vi "generate_chirp_3326A.vi"() -> ()   [LabVIEW 2014]
panel:
  in  "Zero Offsets?":bool=TRUE
  in  "B: Phase (deg)":dbl format="%#_13g"
  in  "A: Phase (deg)":dbl format="%#_13g"
  in  "B: Offset Trim (part per thousand)":i32
  in  "B: Auto Offset":bool=TRUE
  in  "B: Manual Offset (V)":dbl=175.0
  in  "Desired Final Amplitude (V)":dbl format="%#_13g"
  in  "CH B Gain":dbl format="%#_13g"
  in  "CH A Gain":dbl format="%#_13g"
  in  "Step Length (s)":i32=10000
  in  "A: Offset Trim (part per thousand)":i32
  in  "A: Auto Offset":bool=TRUE
  in  "A: Manual Offset (V)":dbl=175.0
  in  "Hz/step":dbl=300.0
  out "Current Freq":dbl format="%#_13g"
  in  "Stop Freq (Hz)":dbl=300.0
  in  "Start Freq (Hz)":dbl=175.0
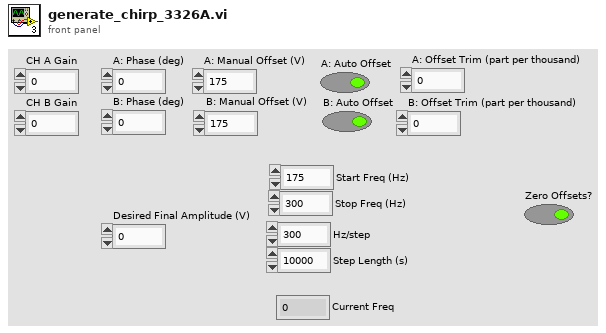
[diagram p1: front panel]
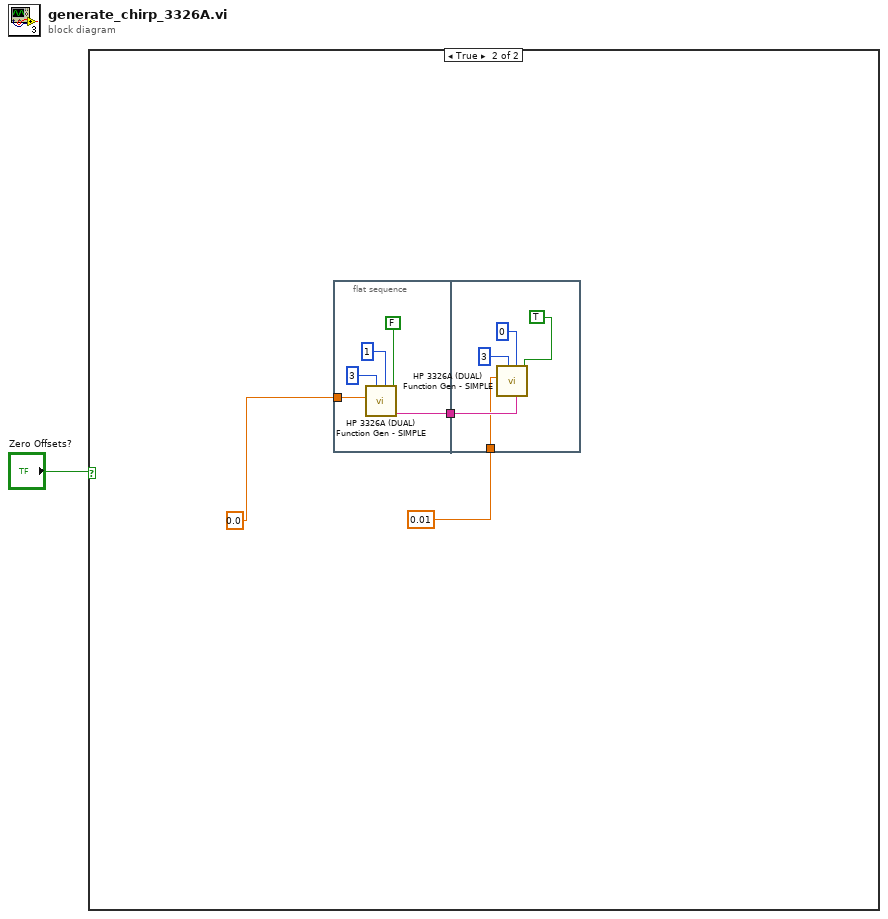
[diagram p0: block diagram]
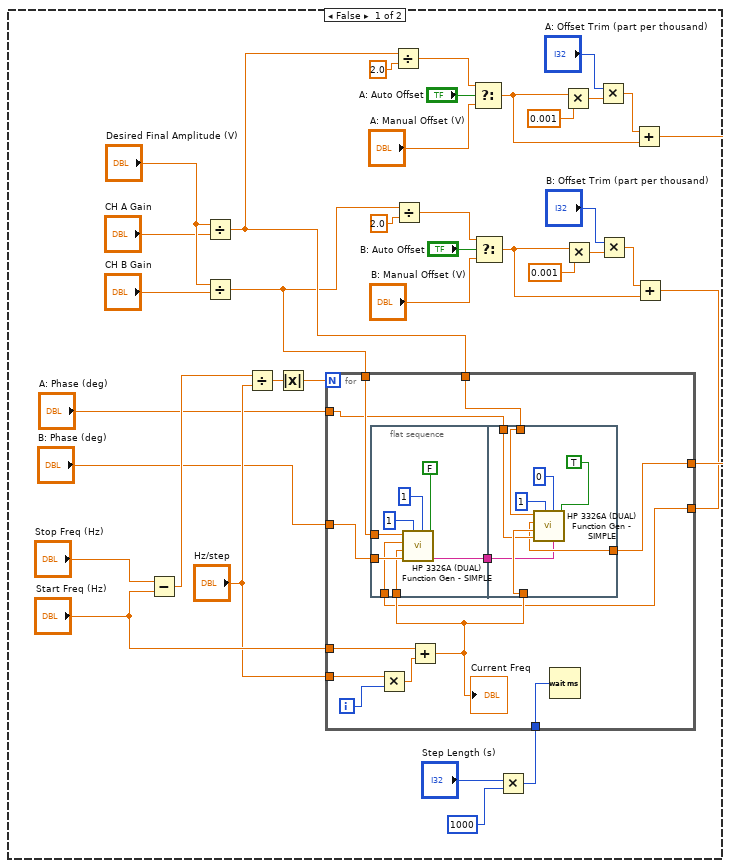
[diagram p2: hidden frame]
diagram:
  n1 = case shown="True" "Zero Offsets?" {
    frame False {
      n2 = Subtract(x="Stop Freq (Hz)", y="Start Freq (Hz)") -> (x-y=w36:dbl)
      n3 = Divide(x="Desired Final Amplitude (V)", y="CH A Gain") -> (x/y=w7:dbl)
      n4 = Divide(x="Desired Final Amplitude (V)", y="CH B Gain") -> (x/y=w6:dbl)
      n5 = Divide(x=w36, y="Hz/step") -> (x/y=w21:dbl)
      n6 = Absolute Value(x=w21) -> (abs(x)=w20:dbl)
      n7 = Divide(x=w7, y=2.0) -> (x/y=w32:dbl)
      n8 = Divide(x=w6, y=2.0) -> (x/y=w14:dbl)
      n9 = Select(t=w32, s="A: Auto Offset", f="A: Manual Offset (V)") -> (s? t:f=w30:dbl)
      n10 = Select(t=w14, s="B: Auto Offset", f="B: Manual Offset (V)") -> (s? t:f=w12:dbl)
      n11 = Multiply(x="Step Length (s)", y=1000) -> (x*y=w22:i32)
      n12 = Multiply(x=w30, y=0.001) -> (x*y=w27:dbl)
      n13 = Multiply(x=w12, y=0.001) -> (x*y=w9:dbl)
      n14 = Multiply(x="A: Offset Trim (part per thousand)", y=w27) -> (x*y=w26:dbl)
      n15 = Multiply(x="B: Offset Trim (part per thousand)", y=w9) -> (x*y=w8:dbl)
      n16 = Add(x=w26, y=w30) -> (x+y=w5:dbl)
      n17 = Add(x=w8, y=w12) -> (x+y=w4:dbl)
      n18 = for {
        N: w20 -> [_]
        tunnel: "Start Freq (Hz)" -> [w49]
        tunnel: "Hz/step" -> [w50]
        tunnel: w22 -> [w46]
        tunnel: w7 -> [w43]
        tunnel: w6 -> [w45]
        tunnel: w5 -> [w40]
        tunnel: w4 -> [w39]
        tunnel: "A: Phase (deg)" -> [w41]
        tunnel: "B: Phase (deg)" -> [w44]
        i -> [w47]
        n19 = flat-sequence {
          tunnel: w45 -> [w57]
          tunnel: w44 -> [w56]
          tunnel: w42 -> [w54]
          tunnel: w39 -> [w53]
          tunnel: [w51] -> w38
          tunnel: w43 -> [w64]
          tunnel: w42 -> [w63]
          tunnel: w41 -> [w62]
          tunnel: w40 -> [w61]
          tunnel: w38 -> [w59]
          frame #0 {
            n20 = call "HP 3326A (DUAL) Function Gen - SIMPLE.vi"("Execute?"=FALSE, "Channel (0:A, 1:B)"=1, "signal type (off:0)"=1, "Phase (deg)"=w56, "frequency (Hz)"=w54, "offset (V)"=w53, "amplitude (V)"=w57) -> ("cmd"=w51:string)  [unwired: 4 in]
          }
          frame #1 {
            n21 = call "HP 3326A (DUAL) Function Gen - SIMPLE.vi"("Execute?"=TRUE, "init cmd"=w59, "Channel (0:A, 1:B)"=0, "signal type (off:0)"=1, "Phase (deg)"=w62, "frequency (Hz)"=w63, "offset (V)"=w61, "amplitude (V)"=w64) -> ()  [unwired: 3 in, 1 out]
          }
        }
        n22 = Multiply(x=w50, y=w47) -> (x*y=w48:dbl)
        n23 = Add(x=w49, y=w48) -> (x+y=w42:dbl)
        "Current Freq" <- w42
        n24 = Wait (ms)(milliseconds to wait=w46) -> ()  [unwired: 1 out]
      }
    }
    frame True {
      n25 = flat-sequence {
        tunnel: [w71] -> w69
        tunnel: 0.0 -> [w70]
        tunnel: w69 -> [w76]
        tunnel: 0.01 -> [w75]
        frame #0 {
          n26 = call "HP 3326A (DUAL) Function Gen - SIMPLE.vi"("Execute?"=FALSE, "Channel (0:A, 1:B)"=1, "signal type (off:0)"=3, "offset (V)"=w70) -> ("cmd"=w71:string)  [unwired: 7 in]
        }
        frame #1 {
          n27 = call "HP 3326A (DUAL) Function Gen - SIMPLE.vi"("Execute?"=TRUE, "init cmd"=w76, "Channel (0:A, 1:B)"=0, "signal type (off:0)"=3, "offset (V)"=w75) -> ()  [unwired: 6 in, 1 out]
        }
      }
    }
  }
